vi "IFD U16 Image in.vi"(8 "error in (no error)":errorcluster, 10 "U16 Array":u16[][](array[numeric]), 11 "IFD in":refnum<class "IFD.lvclass">) -> (0 "error out":errorcluster, 3 "IFD out":refnum<class "IFD.lvclass">)   [LabVIEW 2016, in "IFD.lvclass"]
uses:
  IFD.lvclass
  IFD.lvclass/IFD.ctl
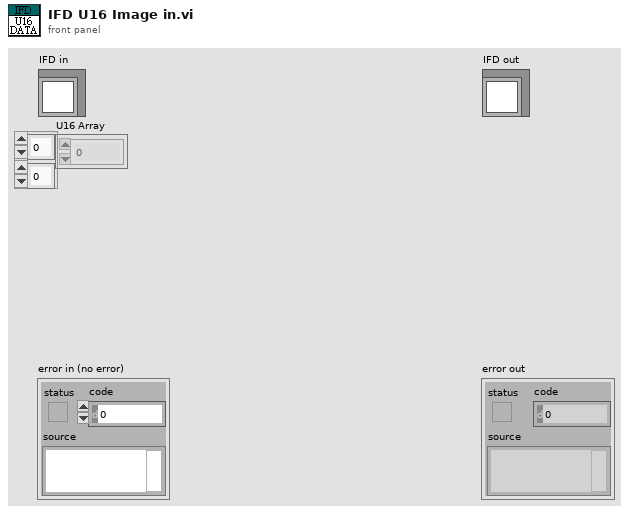
[diagram p1: front panel]
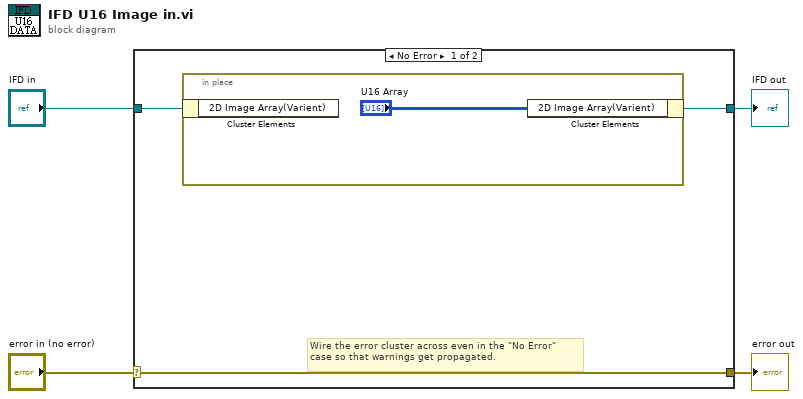
[diagram p0: block diagram]
diagram:
  n1 = case shown="No Error" "error in (no error)" {
    selector: "error in (no error)" -> [w7 w10]
    tunnel: [w7 w10] -> w3
    tunnel: [w5 w9] -> w1
    tunnel: "IFD in" -> [w6 w9]
    frame No Error {
      # "Wire the error cluster across even in the \"No Error\"\ncase so that warnings get propagated."
      n2 = in-place {
        n3 = in-place-cluster #1(w6) -> ()  [unwired: 1 out]
        n4 = in-place-cluster #1("2D Image Array(Varient)"="U16 Array") -> (w5:refnum<class "IFD.lvclass">)
      }
    }
    frame Error {
    }
  }
  "error out" <- w3
  "IFD out" <- w1
